vi "3-4.vi"(10 "参考电压Vref（V）":dbl=2.56, 11 "模拟信号参数":cluster{"频率(Hz)":dbl, "幅值(V)":dbl}={"频率(Hz)"=100.0, "幅值(V)"=2.5}) -> (1 "信噪比(dB)":dbl, 2 "量化噪声":waveform(dbl)(graph), 3 "复原信号":waveform(dbl)(graph))   [LabVIEW 2018]
uses:
  <vilib>/measure/NI_MABase.lvlib
panel:
  out "噪声平均功率":dbl
  out "信号平均功率":dbl
  out "输入信号":waveform(dbl)(graph)
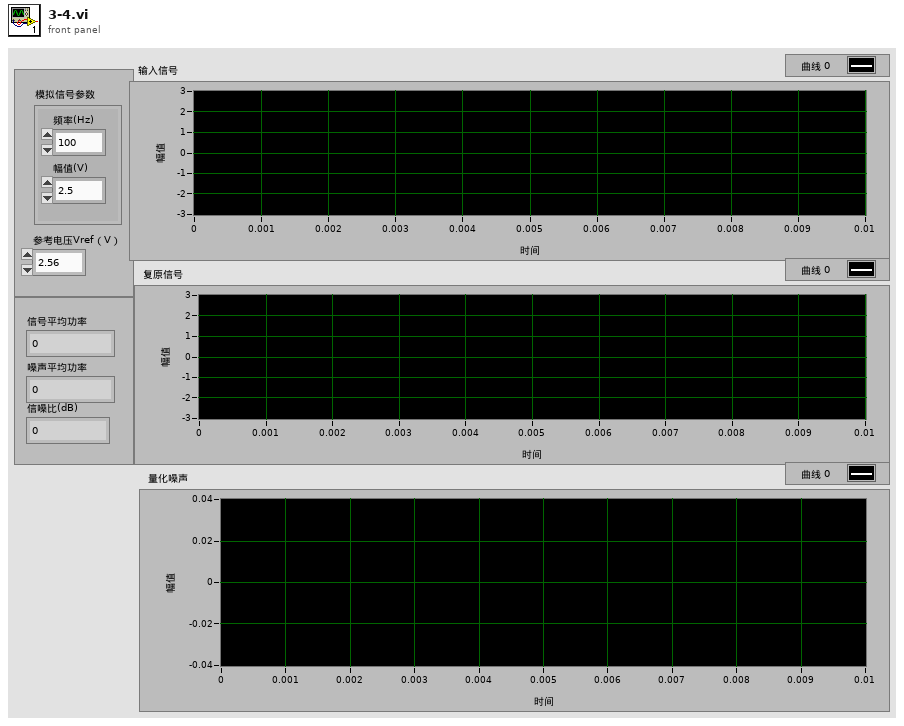
[diagram p1: front panel]
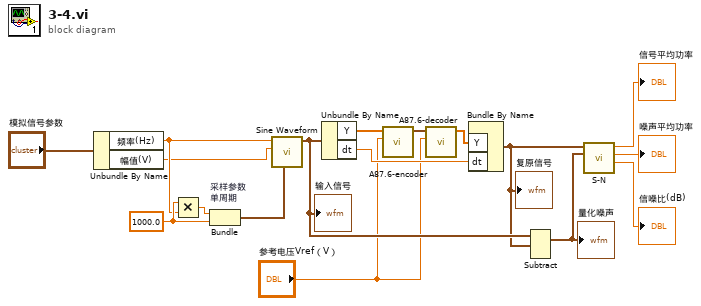
[diagram p0: block diagram]
diagram:
  w15 = 1000.0 ("x")
  n1 = Unbundle By Name("模拟信号参数") -> ("频率(Hz)"=w13:dbl, "幅值(V)"=w12:dbl)
  n2 = Multiply(x=w15, y=w13) -> (x*y=w16:dbl)
  n3 = Bundle "采样参数\n单周期"(w16, "x"=w15) -> (w14:cluster{dbl, "x":dbl})  [unwired: 1 in]
  n4 = call <vilib>:"Sine Waveform.vi"("sampling info"=w14, "amplitude"=w12, "frequency"=w13) -> ("signal out"=w10:waveform(dbl))  [unwired: 7 in, 1 out]
  "输入信号" <- w10
  n5 = Unbundle By Name(w10) -> ("Y"=w4:dbl[], "dt"=w11:dbl)
  n6 = call "A87.6-encoder.vi"("参考电压Vref（V）"="参考电压Vref（V）", "信号数组"=w4) -> ("编码数组"=w3:digitaldata)  [unwired: 9 in]
  n7 = call "A87.6-decoder.vi"("参考电压（V）"="参考电压Vref（V）", "编码数组"=w3) -> ("还原信号数组"=w1:dbl[])  [unwired: 9 in]
  n8 = Bundle By Name("Y"=w1, "dt"=w11) -> (w9:waveform(dbl))  [unwired: 1 in]
  "复原信号" <- w9
  n9 = Subtract(1:w9, 2:w10) -> (0:w8:waveform(dbl))  [unwired: 1 in, 1 out]
  "量化噪声" <- w8
  n10 = call "S-N.vi"("signal in 2"=w8, "signal in"=w9) -> ("信噪比(dB)"=→"信噪比(dB)":dbl, "噪声平均功率"=→"噪声平均功率":dbl, "信号平均功率"=→"信号平均功率":dbl)  [unwired: 7 in]
